vi "datatakersync_master.vi"() -> ()   [LabVIEW 2013, in "filenames.lvlib"]
doc: "This example demonstrates how to acquire a single buffer of voltage measurements using a DAQmx device.\n\nFor instructions on how to connect your signals to the DAQ device, refer to your device documentation."
uses:
  filenames.lvlib
  <vilib>/Analysis/3filter.llb/Filter Passband Type.ctl
  <vilib>/Utility/error.llb/DialogType.ctl
  <vilib>/DAQmx/write.llb/DAQmx Write (Analog 1D DBL 1Chan NSamp).vi
  <userlib>/Agilis Labview 7.1/AGILIS.llb/enter / leave remote mode.vi
  <vilib>/LabVIEW Hacker/LINX/Public/Peripherals/Analog/Analog Read 1 Chan.vi
  <vilib>/DAQmx/create/channels.llb/DAQmx Create Channel (AO-Voltage-Basic).vi
  <vilib>/DAQmx/configure/timing.llb/DAQmx Timing (Sample Clock).vi
  <vilib>/DAQmx/create/channels.llb/DAQmx Create Channel (AI-Voltage-Basic).vi
  <vilib>/DAQmx/configure/trigger.llb/DAQmx Start Trigger (Digital Edge).vi
  <vilib>/DAQmx/miscellaneous.llb/DAQmx Fill In Error Info.vi
  <resource>/objmgr/daqmx.rc
  <vilib>/LabVIEW Hacker/LINX/LVH-LINX.lvlib
  <vilib>/ptbypt/NI_PtbyPt.lvlib
  <vilib>/Analysis/NI_AALBase.lvlib
panel:
  in  "Jog during auto":bool=TRUE
  in  "Move Slide Back 3":bool
  in  "Move Slide  2":bool
  in  "Slide Jog Speed 2":i32(slide) scale=1.0..3.0
  in  "Stop Button":bool=TRUE
  in  "Use interferometer":bool=TRUE
  out "Motion Direction Indicator":bool
  out "Move Indicator":bool
  in  "Auto Move":bool=TRUE
  in  "Auto Motion Direction":bool
  in  "Tab Control":T1(tab)=enum."I/O"
  out "Indicator Pos 2":bool
  out "Indicator Pos 1":bool=TRUE
  in  "Go to 2":bool
  in  "Go to 1":bool
  in  "Cycles Between Movements":i32=1
  in  "Position 2":dbl=2.5
  in  "Position 1":dbl=-2.5
  out "Main Sig":dbl[][](graph)=[[-1.679588746006175], [-2.01550649520741]]
  out "Main Output":dbl(graph)=1.3000000000000012
  out "Displacement":dbl=1.3000000000000012 format="%#.3f"
  in  "Zero":bool
  in  "Go to Zero":bool
  in  "Automatic":bool=TRUE
  in  "Motion Direction":bool=TRUE
  in  "Manual Move":bool
  in  "Stop Movement":bool
  in  "Arduino Serial Port":refnum<visa-resource-name>="COM3"
  out "Device Name":string="Arduino Mega 2560"
  in  "Analog Channel":u8
  out "Filtered Signal":dbl(graph)=-1.679588746006175
  in  "filter type":T2=enum."Bandpass"
  in  "order":i32=2
  in  "initialize":bool
  in  "low cutoff freq: fl":dbl=0.45 format="%#_13g"
  out "Raw Signal":dbl(graph)=2.294921875
  in  "Positive Move Steps":i32=30
  in  "Controller Serial Port":u8=6
  in  "Negative Move Steps":i32=30
  in  "Move Period (ms)":u32=10
  in  "high cutoff freq: fh":dbl=1.0
  out "Input Signals":dbl[][](graph)=[[-1.679588746006175], [-2.01550649520741]]
  out "Stepped Signal":dbl(graph)=2.0
  in  "Fringe Counter Settings":T3={"Wavelength"=3.25e-07, "Divisions"=2.0, "Scaling Amplitude"=1.2, "Scaling Offset"=0.0} {"Scaling Offset" format="%0.2f"; "Scaling Amplitude" format="%0.2f"}
  out "Fringe Counter Output Signal":dbl[](graph)=[1.21875e-06]
  out "Relative Displacement":dbl=1.21875e-06
  out "Total Displacement":dbl(graph)=1.3000000000000012
  out "Reset Fringe Counter":bool
  out "Timeout":bool
  in  "Slide Jog Speed":i32(slide) scale=1.0..3.0
  in  "Move Slide":bool
  in  "Move Slide Back":bool
  in  "Error In":errorcluster
  in  "Turn off drive\nwhen flashing?":bool
  in  "set synth":bool
  in  "Sweep type":u16(ring)=1 items=["Chirp", "Single freq", "Both"]
  in  "VISA session":refnum<visa-resource-name>="GPIB0::10::INSTR"
  in  "Physical Channel synth_trigger":tag="Dev5/ao0"
  in  "Digitize on\nother comp?":bool
  in  "stop (F)":ext=100.0
  in  "start (F)":ext=100.0
  in  "Number of F Steps":i32=1
  in  "dc offset?":bool
  in  "volt_div":dbl=200.0
  in  "stop (V)":ext=0.05
  in  "start (V)":ext=0.05
  in  "Number of V Steps":i32=1
  out "error out":errorcluster
  in  "Physical Channel (drive signals)":tag="Dev5/ai0"
  out "Curr threshold":dbl
  in  "Stop threshold":dbl=0.05
  in  "Stop flashing below thresh":bool
  out "Pirani pressure (mbar)":string
  out "CC read error":errorcluster={"status"=FALSE, "code"=1073676294, "source"="VISA Read in read_pressure(SubVI).vi->hdf5(SubVI).vi->filenames.lvlib:datatakersync_master.vi"}
  out "CC pressure (mbar)":string
  out "Pirani read error":errorcluster={"status"=FALSE, "code"=1073676294, "source"="VISA Read in read_pressure(SubVI).vi->hdf5(SubVI).vi->filenames.lvlib:datatakersync_master.vi"}
  in  "# Pulses":i32=3
  in  "Output channel (for flashing)":tag="Dev4/ao0"
  in  "Number of cyles\nbetween flashes":i32=3
  in  "Flash lamp?":bool
  in  "File base name":string="urmbar_xyzcool_close"
  in  "Delay time between files(s)":dbl caption="Delay Time (s)"
  in  "Num files":i32=1000
  out "Temps (C):":dbl[](array[numeric])
  in  "VISA Refnum in":refnum<visa-resource-name>="GPIB0::19::INSTR"
  in  "Directory path":path=path "D:/Data/20150331/Bead6/tapping_close2"
  out "Waveform Graph":dbl[][](graph)
  in  "Number of Samples":i32=1000
  in  "Sample Rate":dbl=10000.0
  in  "Sample Clock Source":tag="/Dev2/PXI_Clk10"
  in  "Terminal Configuration":i32(ring)=-1 items=["default"=-1, "RSE"=10083, "NRSE"=10078, "Differential"=10106, "Pseudodifferential"=12529]
  in  "Max Voltage":dbl=10.0
  in  "Physical Channels (Position signals)":tag="Dev2/ai0:7"
  out "Actual Sample Rate":dbl=10000.0 format="%0.2f"
  # "Channel Settings"
  # "Acquired Data"
  # "Timing Settings"
  # "Flash Lamp Settings"
  # "Pressures and Temperatures"
  # "Logging Settings"
  # "."
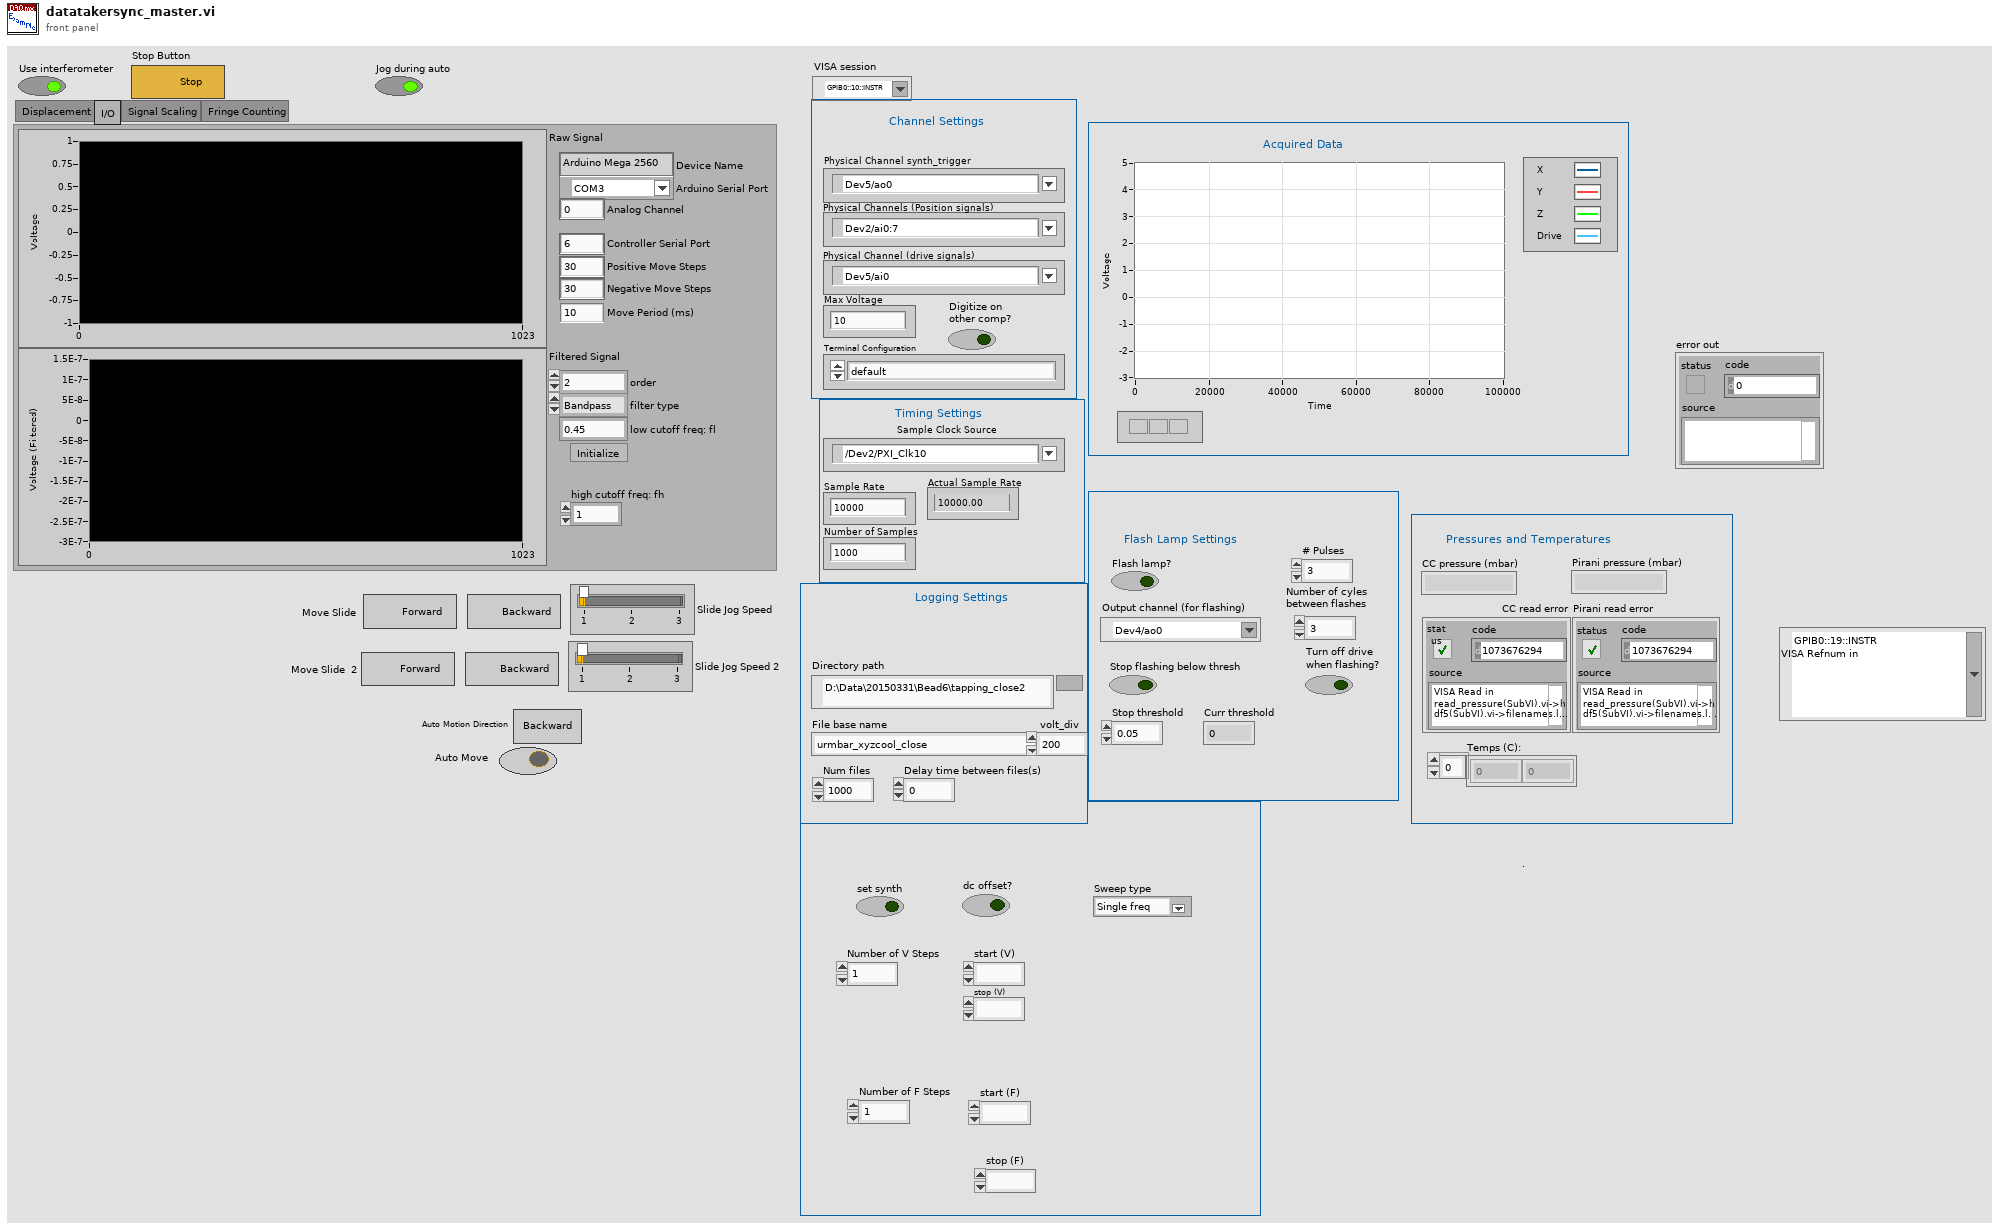
[diagram p1: front panel]
types:
  T1 = enum32{"Displacement", "I/O", "Signal Scaling", "Fringe Counting"}
  T2 = typedef "NI_AALBase.lvlib/Filter Passband Type.ctl" = enum32{"Lowpass", "Highpass", "Bandpass", "Bandstop"}
  T3 = cluster{"Wavelength":dbl, "Divisions":dbl, "Scaling Amplitude":dbl, "Scaling Offset":dbl}
  T4 = typedef "DialogType.ctl" = u16
  T5 = typedef "LVH-LINX.lvlib/LINX Ref.ctl" = cluster{"Platform":T6, "Interface":T7, "LINX Device Config":T8}
  T6 = typedef "LVH-LINX.lvlib/Platform.ctl" = enum16{"LINX", "myRIO"}
  T7 = typedef "LVH-LINX.lvlib/Interface.ctl" = enum16{"Serial", "TCP"}
  T8 = typedef "LVH-LINX.lvlib/Device.lvlib/LINX Device Config.ctl" = cluster{"Interface":T7, "COM Port":refnum<visa-resource-name>, "TCP Configuration":T9, "Device Family":T10, "Device ID":u8, "Device Name":string, "TCP Ref":refnum<k5>}
  T9 = typedef "LVH-LINX.lvlib/Device.lvlib/TCP Config.ctl" = cluster{"IP Address":string, "Port":u16}
  T10 = typedef "LVH-LINX.lvlib/Device Family.ctl" = enum8{"National Instruments", "Digilent", "Arduino"}
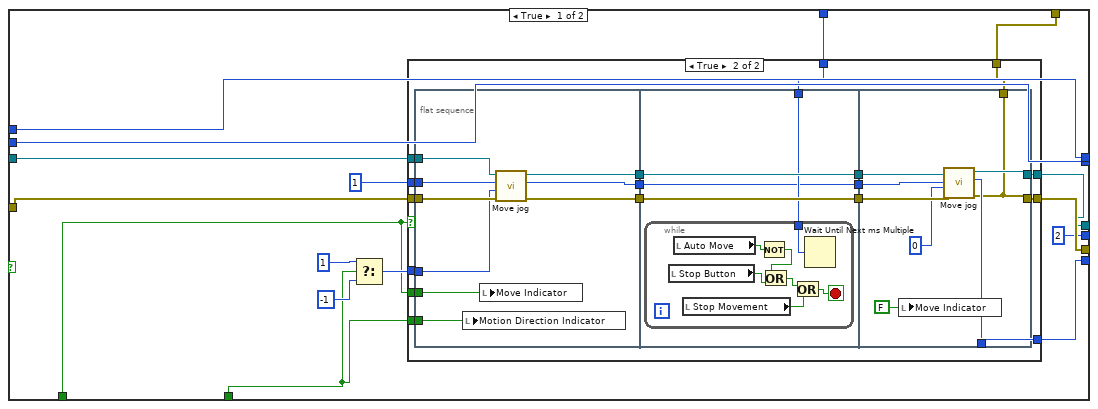
[diagram p3: hidden frame]
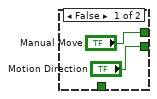
[diagram p5: hidden frame]
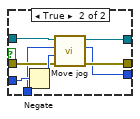
[diagram p6: hidden frame]
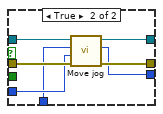
[diagram p7: hidden frame]
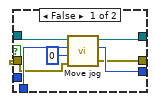
[diagram p8: hidden frame]
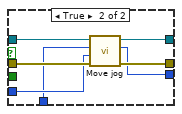
[diagram p9: hidden frame]
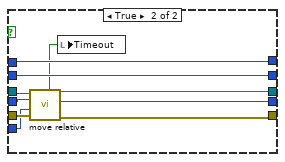
[diagram p10: hidden frame]
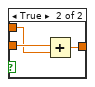
[diagram p13: hidden frame]
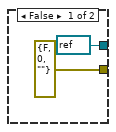
[diagram p14: hidden frame]
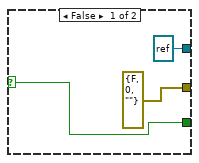
[diagram p17: hidden frame]
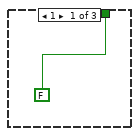
[diagram p18: hidden frame]
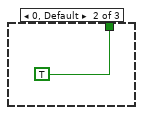
[diagram p19: hidden frame]
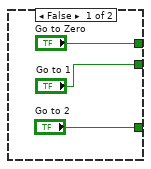
[diagram p20: hidden frame]
diagram:
  w10 = TRUE  # ID Query
  w46 = 10178 items=["Finite Samples"=10178, "Continuous Samples"=10123, "Hardware Timed Single Point"=12522]  # Sample Mode
  n1 = case shown="True" "set synth" {
    tunnel: w10 -> [_ w54]
    tunnel: [refnum<visa-resource-name> refnum ("dup VISA session") w51] -> w9
    tunnel: [errorcluster {"status"=FALSE, "code"=0, "source"=""} ("error out") w50] -> w8
    frame False {
    }
    frame True {
      n2 = call <vilib>:"ag33xxx - Initialize.vi"("ID Query (T: Check)"=w54, "Instrument Resource Name"="VISA session") -> ("error out"=w53:errorcluster, "dup VISA session"=w52:refnum<visa-resource-name>)  [unwired: 8 in]
      n3 = VISA Write(VISA resource name=w52, write buffer="SOUR:BM:NCYC INF;:SOUR:BM:PHAS 0;SOUR INT;:TRIG:SOUR EXT;:SOUR:BM:INT:RATE 1.000000;:BM:STAT ON;", error in (no error)=w53) -> (VISA resource name out=w51:refnum<visa-resource-name>, error out=w50:errorcluster)  [unwired: 1 out]
    }
  }
  n4 = call <vilib>:"Check if File or Folder Exists.vi"("path"="Directory path") -> ("file or folder exists?"=w36:bool, "dup path"=w35:path)  [unwired: 8 in, 1 out]
  n5 = case shown="False" w36 {
    tunnel: w35 -> [w57 w62]
    tunnel: [w56 w62] -> w34
    frame False {
      n6 = flat-sequence {
        tunnel: w57 -> [w61]
        tunnel: [w60] -> w56
        frame #0 {
          n7 = call "Create folder?"() -> ("OK"=w59:bool)  [unwired: 18 in, 1 out]
          n8 = Not(x=w59) -> (.not. x?=w58:bool)
          n9 = Stop(stop? (T)=w58) -> ()
        }
        frame #1 {
          n10 = Create Folder(path (use dialog)=w61) -> (created path=w60:path)  [unwired: 2 in, 2 out]
        }
      }
    }
    frame True {
    }
  }
  n11 = Subtract(x="stop (F)", y="start (F)") -> (x-y=w22:ext)
  n12 = Divide(x=w22, y="Number of F Steps") -> (x/y=w21:ext)
  n13 = Subtract(x="stop (V)", y="start (V)") -> (x-y=w29:ext)
  n14 = Multiply(x="Max Voltage", y=-1.0) -> (x*y=w39:dbl)
  n15 = Divide(x=w29, y="Number of V Steps") -> (x/y=w27:ext)
  n16 = case shown="True" "Digitize on\nother comp?" {
    selector: "Digitize on\nother comp?" -> [w63 w66]
    tunnel: [errorcluster {"status"=FALSE, "code"=0, "source"=""} ("error out") w69] -> w18
    tunnel: [refnum<k5> refnum ("connection ID") w68] -> w17
    tunnel: [w63 w66] -> w13
    frame False {
    }
    frame True {
      w70 = 60000  # timeout ms
      n17 = call <vilib>:"TCP Listen.vi"("timeout ms (wait forever: -1)"=w70, "port"=u16 6340) -> ("error out"=w69:errorcluster, "connection ID"=w68:refnum<k5>)  [unwired: 5 in, 3 out]
    }
  }
  n18 = local write "Automatic"(FALSE ("Go to Zero")) -> ()
  n19 = for {
    N: "Num files" -> [_]
    tunnel: w46 -> [w107]
    tunnel: "Physical Channels (Position signals)" -> [w106]
    tunnel: "Terminal Configuration" -> [w105]
    tunnel: "Sample Clock Source" -> [w104]
    tunnel: "Sample Rate" -> [w103]
    tunnel: "Number of Samples" -> [w102]
    tunnel: w39 -> [w101]
    tunnel: "Max Voltage" -> [w100]
    tunnel: w34 -> [w99]
    tunnel: "File base name" -> [w98]
    tunnel: "Output channel (for flashing)" -> [w97]
    tunnel: "Physical Channel (drive signals)" -> [w96]
    tunnel: "Number of V Steps" -> [w95]
    tunnel: w27 -> [w94]
    tunnel: "start (V)" -> [w93]
    tunnel: "Num files" -> [w92]
    tunnel: "set synth" -> [w91]
    tunnel: "volt_div" -> [w90]
    tunnel: w21 -> [w89]
    tunnel: "start (F)" -> [w88]
    tunnel: "Number of F Steps" -> [w87]
    tunnel: w18 -> [w86]
    tunnel: w17 -> [w85]
    tunnel: [w84] -> w16
    tunnel: [w83] -> w15
    tunnel: w13 -> [w82]
    tunnel: [w81] -> w12
    tunnel: "Physical Channel synth_trigger" -> [w80]
    tunnel: w9 -> [w79]
    tunnel: w8 -> [w78]
    tunnel: [w77] -> w7
    tunnel: [w76] -> w6
    tunnel: [w75] -> w5
    tunnel: "set synth" -> [w74]
    tunnel: "Sweep type" -> [w72]
    i -> [w71]
    n20 = case shown="2" w72 {
      tunnel: [FALSE TRUE w110] -> w73
      tunnel: w71 -> [_ _ w114]
      frame 1 {
      }
      frame 0, Default {
      }
      frame 2 {
        n21 = Quotient & Remainder(x=w114, y=2) -> (x-y*floor(x/y)=w112:i32)  [unwired: 1 out]
        n22 = Equal?(x=w112, y=0) -> (x = y?=w110:bool)
      }
    }
    n23 = for {
      N: w95 -> [_]
      tunnel: w107 -> [w151]
      tunnel: w106 -> [w150]
      tunnel: w105 -> [w149]
      tunnel: w104 -> [w148]
      tunnel: w103 -> [w147]
      tunnel: w102 -> [w146]
      tunnel: w101 -> [w145]
      tunnel: w100 -> [w144]
      tunnel: w99 -> [w143]
      tunnel: w98 -> [w142]
      tunnel: w97 -> [w141]
      tunnel: w96 -> [w140]
      tunnel: w94 -> [w139]
      tunnel: w93 -> [w138]
      tunnel: w71 -> [w136]
      tunnel: w92 -> [w135]
      tunnel: w91 -> [w134]
      tunnel: w90 -> [w133]
      tunnel: w89 -> [w132]
      tunnel: w88 -> [w131]
      tunnel: w87 -> [w130]
      tunnel: w73 -> [w129]
      tunnel: w86 -> [w128]
      tunnel: w85 -> [w127]
      tunnel: [w126] -> w84
      tunnel: [w125] -> w83
      tunnel: w82 -> [w124]
      tunnel: [w123] -> w81
      tunnel: w80 -> [w122]
      tunnel: w79 -> [w121]
      tunnel: w78 -> [w120]
      tunnel: [w119] -> w77
      tunnel: [w118] -> w76
      tunnel: [w117] -> w75
      tunnel: w74 -> [w116]
      tunnel: w71 -> [w115]
      i -> [w137]
      n24 = for {
        N: w130 -> [_]
        tunnel: w151 -> [w284]
        tunnel: w150 -> [w283]
        tunnel: w149 -> [w282]
        tunnel: w148 -> [w281]
        tunnel: w147 -> [w209]
        tunnel: w146 -> [w280]
        tunnel: w145 -> [w279]
        tunnel: w144 -> [w278]
        tunnel: w143 -> [w277]
        tunnel: w142 -> [w276]
        tunnel: w141 -> [w275]
        tunnel: w140 -> [w274]
        tunnel: w139 -> [w273]
        tunnel: w138 -> [w271]
        tunnel: w137 -> [w269]
        tunnel: w136 -> [w268]
        tunnel: w135 -> [w237]
        tunnel: w134 -> [w267]
        tunnel: w133 -> [w266]
        tunnel: w132 -> [w262]
        tunnel: w131 -> [w261]
        tunnel: w129 -> [w259]
        tunnel: w128 -> [w258]
        tunnel: w127 -> [w257]
        tunnel: [w256] -> w126
        tunnel: [w255] -> w125
        tunnel: w124 -> [w254]
        tunnel: [w253] -> w123
        tunnel: w122 -> [w208]
        tunnel: w121 -> [w204]
        tunnel: w120 -> [w203]
        tunnel: [w199] -> w119
        tunnel: [w195] -> w118
        tunnel: [w194] -> w117
        tunnel: w116 -> [w190]
        tunnel: w115 -> [w152]
        i -> [w260]
        n25 = Multiply(x=w262, y=w260) -> (x*y=w263:ext)
        n26 = Add(x=w261, y=w263) -> (x+y=w264:ext)
        n27 = Multiply(x=w269, y=w273) -> (x*y=w272:ext)
        n28 = Add(x=w271, y=w272) -> (x+y=w270:ext)
        n29 = flat-sequence {
          tunnel: w190 -> [w292]
          tunnel: w203 -> [w293]
          tunnel: w204 -> [w294]
          tunnel: w208 -> [w295]
          tunnel: w254 -> [w296]
          tunnel: w257 -> [w297]
          tunnel: w258 -> [w298]
          tunnel: w259 -> [w299]
          tunnel: "dc offset?" -> [w300]
          tunnel: w267 -> [w301]
          tunnel: w268 -> [w302]
          tunnel: w270 -> [w303]
          tunnel: w270 -> [w304]
          tunnel: w264 -> [w305]
          tunnel: w274 -> [w306]
          tunnel: w275 -> [w307]
          tunnel: w276 -> [w308]
          tunnel: w277 -> [w309]
          tunnel: w278 -> [w310]
          tunnel: w279 -> [w311]
          tunnel: w281 -> [w312]
          tunnel: w282 -> [w313]
          tunnel: w283 -> [w314]
          tunnel: [w314] -> w175
          tunnel: [w313] -> w174
          tunnel: [w312] -> w173
          tunnel: [w311] -> w172
          tunnel: [w310] -> w171
          tunnel: [w309] -> w170
          tunnel: [w308] -> w169
          tunnel: [w307] -> w168
          tunnel: [w306] -> w167
          tunnel: [w305] -> w166
          tunnel: [w304] -> w165
          tunnel: [w303] -> w164
          tunnel: [w302] -> w163
          tunnel: [w301] -> w162
          tunnel: [w300] -> w161
          tunnel: [w299] -> w160
          tunnel: [w298] -> w159
          tunnel: [w297] -> w158
          tunnel: [w296] -> w157
          tunnel: [w295] -> w156
          tunnel: [w294] -> w155
          tunnel: [w293] -> w154
          tunnel: [w292] -> w153
          tunnel: w152 -> [w285]
          tunnel: [w391] -> w241
          tunnel: [w390] -> w242
          tunnel: [w389] -> w243
          tunnel: [w388] -> w244
          tunnel: [w387] -> w245
          tunnel: [w386] -> w246
          tunnel: [w385] -> w247
          tunnel: [w384] -> w248
          tunnel: [w383] -> w249
          tunnel: [w381] -> w250
          tunnel: [w380] -> w251
          tunnel: [w379] -> w252
          tunnel: [w377] -> w240
          tunnel: [w376] -> w239
          tunnel: [w375] -> w238
          tunnel: [w374] -> w207
          tunnel: [w371] -> w202
          tunnel: [w370] -> w198
          tunnel: [w369] -> w191
          tunnel: [w368] -> w186
          tunnel: [w367] -> w185
          tunnel: [w366] -> w180
          tunnel: w175 -> [w391]
          tunnel: w174 -> [w390]
          tunnel: w173 -> [w389]
          tunnel: w172 -> [w388]
          tunnel: w171 -> [w387]
          tunnel: w170 -> [w386]
          tunnel: w169 -> [w385]
          tunnel: w168 -> [w384]
          tunnel: w167 -> [w383]
          tunnel: w166 -> [w381]
          tunnel: w165 -> [w382]
          tunnel: w164 -> [w380]
          tunnel: w163 -> [w379]
          tunnel: w162 -> [w378]
          tunnel: w161 -> [w366]
          tunnel: w160 -> [w368]
          tunnel: w159 -> [w377]
          tunnel: w158 -> [w376]
          tunnel: w157 -> [w375]
          tunnel: w156 -> [w374]
          tunnel: w155 -> [w373]
          tunnel: w154 -> [w372]
          tunnel: w153 -> [w369]
          tunnel: w252 -> [w443]
          tunnel: w251 -> [w413]
          tunnel: w250 -> [w448]
          tunnel: [w448] -> w236
          tunnel: w249 -> [w457]
          tunnel: [w457] -> w234
          tunnel: w248 -> [w456]
          tunnel: [w456] -> w232
          tunnel: w247 -> [w422]
          tunnel: w246 -> [w424]
          tunnel: w245 -> [w455]
          tunnel: [w455] -> w229
          tunnel: w244 -> [w454]
          tunnel: [w454] -> w227
          tunnel: w243 -> [w453]
          tunnel: [w453] -> w225
          tunnel: w242 -> [w452]
          tunnel: [w452] -> w223
          tunnel: w241 -> [w451]
          tunnel: [w451] -> w221
          tunnel: w240 -> [w433]
          tunnel: [w430] -> w219
          tunnel: w239 -> [w434]
          tunnel: [w431] -> w217
          tunnel: w238 -> [w432]
          tunnel: [w429] -> w215
          tunnel: [w449] -> w213
          tunnel: w237 -> [w446]
          tunnel: [w443] -> w211
          tunnel: w207 -> [w428]
          tunnel: [w428] -> w205
          tunnel: w202 -> [w427]
          tunnel: [w427] -> w200
          tunnel: w198 -> [w426]
          tunnel: [w426] -> w196
          tunnel: [w425] -> w193
          tunnel: w191 -> [w425]
          tunnel: [w424] -> w189
          tunnel: [w423] -> w188
          tunnel: w186 -> [w416]
          tunnel: w185 -> [w415]
          tunnel: [w416] -> w183
          tunnel: [w415] -> w182
          tunnel: w180 -> [w414]
          tunnel: [w414] -> w179
          tunnel: [w413] -> w177
          tunnel: w236 -> [w515]
          tunnel: [w515] -> w235
          tunnel: w234 -> [w514]
          tunnel: [w514] -> w233
          tunnel: w232 -> [w513]
          tunnel: [w513] -> w231
          tunnel: [w512] -> w230
          tunnel: w229 -> [w511]
          tunnel: [w511] -> w228
          tunnel: w227 -> [w510]
          tunnel: [w510] -> w226
          tunnel: w225 -> [w509]
          tunnel: [w509] -> w224
          tunnel: w223 -> [w508]
          tunnel: [w508] -> w222
          tunnel: w221 -> [w502]
          tunnel: [w502] -> w220
          tunnel: w219 -> [w507]
          tunnel: [w507] -> w218
          tunnel: w217 -> [w506]
          tunnel: [w506] -> w216
          tunnel: w215 -> [w505]
          tunnel: [w505] -> w214
          tunnel: w213 -> [w504]
          tunnel: [w504] -> w212
          tunnel: w211 -> [w503]
          tunnel: [w503] -> w210
          tunnel: [w501] -> w206
          tunnel: w205 -> [w501]
          tunnel: [w500] -> w201
          tunnel: w200 -> [w500]
          tunnel: [w499] -> w197
          tunnel: w196 -> [w499]
          tunnel: w193 -> [w498]
          tunnel: [w498] -> w192
          tunnel: w189 -> [w512]
          tunnel: w188 -> [w497]
          tunnel: [w497] -> w187
          tunnel: [w496] -> w184
          tunnel: w183 -> [w496]
          tunnel: w182 -> [w495]
          tunnel: [w495] -> w181
          tunnel: w179 -> [w494]
          tunnel: [w494] -> w178
          tunnel: w177 -> [w493]
          tunnel: [w493] -> w176
          tunnel: w284 -> [w618]
          tunnel: w209 -> [w538]
          tunnel: w280 -> [w615]
          tunnel: w266 -> [w568]
          tunnel: w235 -> [w528]
          tunnel: w233 -> [w611]
          tunnel: w231 -> [w612]
          tunnel: w230 -> [w562]
          tunnel: w228 -> [w613]
          tunnel: w226 -> [w614]
          tunnel: w224 -> [w560]
          tunnel: w222 -> [w616]
          tunnel: w220 -> [w617]
          tunnel: w218 -> [w564]
          tunnel: w216 -> [w565]
          tunnel: [w564] -> w256
          tunnel: [w565] -> w255
          tunnel: w214 -> [w563]
          tunnel: [w563] -> w253
          tunnel: w212 -> [w567]
          tunnel: w210 -> [w566]
          tunnel: w206 -> [w561]
          tunnel: w201 -> [w523]
          tunnel: [w522] -> w199
          tunnel: w197 -> [w527]
          tunnel: [w521] -> w195
          tunnel: [w546] -> w194
          tunnel: w192 -> [w546]
          tunnel: w187 -> [w545]
          tunnel: w184 -> [w526]
          tunnel: w181 -> [w525]
          tunnel: w178 -> [w524]
          tunnel: w176 -> [w520]
          frame #0 {
            n30 = case shown="True" "Automatic" {
              tunnel: w285 -> [_ w325]
              tunnel: ["Go to Zero" FALSE ("Go to Zero")] -> w288
              tunnel: ["Go to 1" w319] -> w289
              tunnel: ["Go to 2" w320] -> w290
              frame False {
              }
              frame True {
                n31 = Quotient & Remainder(x=w325, y="Cycles Between Movements") -> (x-y*floor(x/y)=w323:i32, floor(x/y)=w321:i32)
                n32 = Equal To 0?(x=w323) -> (x = 0?=w322:bool)
                n33 = case shown="True" w322 {
                  tunnel: w321 -> [_ w331]
                  tunnel: [w326 w328] -> w320
                  tunnel: [w326 w327] -> w319
                  frame False {
                    w326 = FALSE
                  }
                  frame True {
                    n34 = Quotient & Remainder(x=w331, y=2) -> (x-y*floor(x/y)=w329:i32)  [unwired: 1 out]
                    n35 = Equal To 0?(x=w329) -> (x = 0?=w327:bool)
                    n36 = Not(x=w327) -> (.not. x?=w328:bool)
                  }
                }
              }
            }
            n37 = local read "Displacement"() -> (w287:dbl)
            n38 = for {
              N: 3 -> [_]
              tunnel: w288 -> [w337]
              tunnel: w289 -> [w334]
              tunnel: w290 -> [w333]
              tunnel: w287 -> [w335]
              i -> [w338]
              n39 = case shown="2" w338 {
                tunnel: w337 -> [w361 _ _]
                tunnel: w334 -> [_ w363 _]
                tunnel: w333 -> [_ _ w365]
                tunnel: [w361 w363 w365] -> w332
                tunnel: [0.0 ("Position 2") "Position 1" "Position 2"] -> w336
                frame 0, Default {
                }
                frame 1 {
                }
                frame 2 {
                }
              }
              n40 = case shown="True" w332 {
                tunnel: w336 -> [_ w345]
                tunnel: w335 -> [_ w344]
                tunnel: w334 -> [_ w340]
                tunnel: w333 -> [_ w341]
                tunnel: w332 -> [_ w339]
                frame False {
                }
                frame True {
                  n41 = Greater?(x=w345, y=w344) -> (0:w343:bool)
                  n42 = local write "Auto Motion Direction"(w343) -> ()
                  n43 = local write "Auto Move"(w339) -> ()
                  n44 = while {
                    tunnel: w345 -> [w346]
                    tunnel: w343 -> [w358]
                    tunnel: w341 -> [w355]
                    tunnel: w340 -> [w354]
                    tunnel: [FALSE] -> w342
                    stop <- w351 stop-if-true
                    n45 = local read "Displacement"() -> (w347:dbl)
                    n46 = Not Equal?(x=w347, y=w346) -> (x != y?=w348:bool)
                    n47 = Greater?(x=w346, y=w347) -> (0:w359:bool)
                    n48 = Equal?(x=w359, y=w358) -> (x = y?=w353:bool)
                    n49 = And(x=w348, y=w353) -> (x .and. y?=w349:bool)
                    n50 = And(x=w354, y=w349) -> (x .and. y?=→"Indicator Pos 1":bool)
                    n51 = And(x=w355, y=w349) -> (x .and. y?=→"Indicator Pos 2":bool)
                    n52 = Compound Arithmetic op=OR(invert w349, "Stop Movement") -> (w351:bool)
                  }
                  n53 = local write "Auto Move"(w342) -> ()
                }
              }
            }
          }
          frame #1 {
            n54 = case shown="True" w378 {
              tunnel: w382 -> [_ w403]
              tunnel: w381 -> [_ w402]
              tunnel: w366 -> [_ w401]
              tunnel: w368 -> [_ w400]
              tunnel: w373 -> [w393 w399]
              tunnel: w372 -> [w394 w398]
              tunnel: [w394 w397] -> w371
              tunnel: [w393 w396] -> w370
              tunnel: ["no_synth" ("User Def. Wfm Name") w395] -> w367
              frame False {
              }
              frame True {
                n55 = flat-sequence {
                  tunnel: w403 -> [w412]
                  tunnel: w402 -> [w411]
                  tunnel: w401 -> [w410]
                  tunnel: w400 -> [w409]
                  tunnel: w399 -> [w408]
                  tunnel: w398 -> [w407]
                  tunnel: [w406] -> w397
                  tunnel: [w405] -> w396
                  tunnel: [w404] -> w395
                  frame #0 {
                    w404 = "RANDFREQ" ("User Def. Wfm Name")
                    n56 = call "synth_set(SubVI).vi"("dc offset?"=w410, "error in (no error)"=w407, "User Def. Wfm Name"=w404, "chirp?"=w409, "VISA session"=w408, "amplitude (V)"=w412, "frequency (Hz)"=w411) -> ("dup VISA session"=w405:refnum<visa-resource-name>, "error out"=w406:errorcluster)  [unwired: 3 in]
                  }
                  frame #1 {
                    n57 = call "Time Delay2"() -> ()  [unwired: 11 in, 1 out]
                  }
                }
              }
            }
          }
          frame #2 {
            n58 = Multiply(x=w413, y=ext 1000.0) -> (x*y=w449:ext)
            n59 = Number To Decimal String(number=w449) -> (decimal integer string=w420:string)  [unwired: 1 in]
            n60 = Number To Decimal String(number=w448) -> (decimal integer string=w418:string)  [unwired: 1 in]
            n61 = case shown="True" w416 {
              tunnel: [w464 w465] -> w444
              tunnel: w422 -> [w463 w470]
              tunnel: "_" ("string") -> [w462 w469]
              tunnel: w420 -> [w461 w468]
              tunnel: "mV_" ("string") -> [w460 w467]
              tunnel: w418 -> [w459 _]
              tunnel: "Hz" ("string") -> [w458 _]
              tunnel: w415 -> [_ w466]
              frame False {
                n62 = Concatenate Strings(w463, w462, w461, w460, w459, w458) -> (w464:string)
              }
              frame True {
                n63 = Concatenate Strings(w470, w469, w468, w467, w466) -> (w465:string)
              }
            }
            n64 = Greater?(x=w446, y=1) -> (0:w445:bool)
            n65 = case shown="False" w445 {
              tunnel: w443 -> [_ w492]
              tunnel: [w486 w491] -> w442
              tunnel: w444 -> [w485 w490]
              frame False {
                n66 = Concatenate Strings(w485, ".h5" ("string")) -> (w486:string)
              }
              frame True {
                n67 = Number To Decimal String(number=w492) -> (decimal integer string=w488:string)  [unwired: 1 in]
                n68 = Concatenate Strings(w490, "_" ("string"), w488, ".h5" ("string")) -> (w491:string)
              }
            }
            n69 = Build Path(base path=w424, name or relative path=w442) -> (appended path=w423:path)
            n70 = Path To String(path=w423) -> (string=w439:string)
            n71 = Search and Replace String(input string=w439, search string=".h5", replace string="_drive.h5" ("substring (\"\")")) -> (result string=w438:string)  [unwired: 5 in, 3 out]
            n72 = Search and Replace String(input string=w438, search string="D:", replace string="C:" ("replace string (\"\")")) -> (result string=w435:string)  [unwired: 5 in, 3 out]
            n73 = case shown="True" w432 {
              selector: w432 -> [w471 w474]
              tunnel: w433 -> [w472 w483]
              tunnel: w434 -> [w473 w482]
              tunnel: w435 -> [_ w481]
              tunnel: [w472 w476] -> w430
              tunnel: [w473 w475] -> w431
              tunnel: [w471 w474] -> w429
              frame False {
              }
              frame True {
                n74 = String Length(string=w481) -> (length=w478:i32)
                n75 = Type Cast(x=w478) -> (*(type *) &x=w477:string)  [unwired: 1 in]
                n76 = TCP Write(connection ID=w482, data in=w477, error in (no error)=w483) -> (connection ID out=w480:refnum<k5>, error out=w479:errorcluster)  [unwired: 1 in, 1 out]
                n77 = TCP Write(connection ID=w480, data in=w481, error in (no error)=w479) -> (connection ID out=w475:refnum<k5>, error out=w476:errorcluster)  [unwired: 1 in, 1 out]
              }
            }
          }
          frame #3 {
            n78 = call "Time Delay3"() -> ()  [unwired: 11 in, 1 out]
          }
          frame #4 {
            w552 = T4 3 items=["no dialog", "OK message", "continue or stop message", "OK message + warnings", "continue/stop + warnings"] ("type of dialog (OK msg:1)")
            w580 = T4 3 items=["no dialog", "OK message", "continue or stop message", "OK message + warnings", "continue/stop + warnings"] ("type of dialog (OK msg:1)")
            w603 = T4 3 items=["no dialog", "OK message", "continue or stop message", "OK message + warnings", "continue/stop + warnings"] ("type of dialog (OK msg:1)")
            # "Acquire Data"
            # "Acquire Data"
            n79 = flat-sequence {
              tunnel: w538 -> [w644]
              tunnel: w560 -> [w648]
              tunnel: w561 -> [w649]
              tunnel: "# Pulses" -> [w646]
              tunnel: w516 -> [w647]
              tunnel: w611 -> [w650]
              tunnel: w612 -> [w645]
              tunnel: w613 -> [w651]
              tunnel: w614 -> [w652]
              tunnel: w615 -> [w653]
              tunnel: w616 -> [w654]
              tunnel: w617 -> [w655]
              tunnel: [w655] -> w537
              tunnel: [w654] -> w536
              tunnel: [w653] -> w535
              tunnel: [w652] -> w534
              tunnel: [w651] -> w533
              tunnel: [w650] -> w532
              tunnel: [w649] -> w531
              tunnel: [w648] -> w530
              tunnel: [w644] -> w529
              tunnel: w528 -> [w642]
              tunnel: w527 -> [w641]
              tunnel: w526 -> [w640]
              tunnel: w525 -> [w639]
              tunnel: w524 -> [w638]
              tunnel: w523 -> [w637]
              tunnel: [w634] -> w522
              tunnel: [w631] -> w521
              tunnel: w520 -> [w626]
              tunnel: w517 -> [w621]
              tunnel: w618 -> [w751]
              tunnel: [w744] -> w602
              tunnel: [w731] -> w590
              tunnel: [w730] -> w589
              tunnel: [w729] -> w588
              tunnel: [w728] -> w587
              tunnel: [w711] -> w559
              tunnel: [w710] -> w556
              tunnel: w537 -> [w750]
              tunnel: w536 -> [w749]
              tunnel: w535 -> [w748]
              tunnel: w534 -> [w747]
              tunnel: w533 -> [w746]
              tunnel: w532 -> [w745]
              tunnel: w531 -> [w721]
              tunnel: w530 -> [w715]
              tunnel: w529 -> [w709]
              frame #0 {
                n80 = flat-sequence {
                  tunnel: w646 -> [w665]
                  tunnel: [w665] -> w643
                  tunnel: w642 -> [w659]
                  tunnel: w641 -> [w664]
                  tunnel: w640 -> [w660]
                  tunnel: w639 -> [w658]
                  tunnel: w638 -> [w657]
                  tunnel: w637 -> [w663]
                  tunnel: [w662] -> w635
                  tunnel: [w661] -> w632
                  tunnel: [w660] -> w630
                  tunnel: [w659] -> w628
                  tunnel: [w658] -> w625
                  tunnel: [w657] -> w623
                  tunnel: w621 -> [w656]
                  tunnel: [w656] -> w619
                  tunnel: w647 -> [w687]
                  tunnel: w645 -> [w685]
                  tunnel: w644 -> [w684]
                  tunnel: w643 -> [w686]
                  tunnel: [w683] -> w636
                  tunnel: w635 -> [w683]
                  tunnel: [w682] -> w633
                  tunnel: w632 -> [w682]
                  tunnel: w630 -> [w681]
                  tunnel: [w681] -> w629
                  tunnel: w628 -> [w680]
                  tunnel: [w680] -> w627
                  tunnel: w625 -> [w679]
                  tunnel: [w679] -> w624
                  tunnel: w623 -> [w678]
                  tunnel: [w678] -> w622
                  tunnel: [w677] -> w620
                  tunnel: w619 -> [w677]
                  tunnel: w636 -> [w696]
                  tunnel: [w694] -> w634
                  tunnel: w633 -> [w697]
                  tunnel: [w695] -> w631
                  tunnel: w629 -> [w693]
                  tunnel: w627 -> [w692]
                  tunnel: w626 -> [w691]
                  tunnel: w624 -> [w690]
                  tunnel: w622 -> [w689]
                  tunnel: w620 -> [w688]
                  frame #0 {
                    n81 = case shown="True" w656 {
                      tunnel: w664 -> [w667 w675]
                      tunnel: w663 -> [w666 w674]
                      tunnel: [w666 w673] -> w662
                      tunnel: [w667 w672] -> w661
                      tunnel: w660 -> [_ w671]
                      tunnel: w659 -> [_ w670]
                      tunnel: w658 -> [_ w669]
                      tunnel: w657 -> [_ w668]
                      frame False {
                      }
                      frame True {
                        n82 = call "synth_set(SubVI).vi"("dc offset?"=w668, "error in (no error)"=w674, "User Def. Wfm Name"=w669, "chirp?"=w671, "VISA session"=w675, "amplitude (V)"=ext 0.05, "frequency (Hz)"=w670) -> ("dup VISA session"=w672:refnum<visa-resource-name>, "error out"=w673:errorcluster)  [unwired: 3 in]
                        n83 = call "Time Delay4"() -> ()  [unwired: 11 in, 1 out]
                      }
                    }
                  }
                  frame #1 {
                    n84 = call "flasher(SubVI).vi"("Sample Rate"=w684, "# Pulses"=w686, "Boolean"=w687, "Output channel (for flashing)"=w685) -> ()  [unwired: 8 in]
                  }
                  frame #2 {
                    n85 = case shown="True" w688 {
                      tunnel: w697 -> [w698 w708]
                      tunnel: w696 -> [w699 w707]
                      tunnel: [w698 w706] -> w695
                      tunnel: [w699 w705] -> w694
                      tunnel: w693 -> [_ w704]
                      tunnel: w692 -> [_ w703]
                      tunnel: w691 -> [_ w702]
                      tunnel: w690 -> [_ w701]
                      tunnel: w689 -> [_ w700]
                      frame False {
                      }
                      frame True {
                        n86 = call "synth_set(SubVI).vi"("dc offset?"=w700, "error in (no error)"=w707, "User Def. Wfm Name"=w701, "chirp?"=w704, "VISA session"=w708, "amplitude (V)"=w702, "frequency (Hz)"=w703) -> ("dup VISA session"=w706:refnum<visa-resource-name>, "error out"=w705:errorcluster)  [unwired: 3 in]
                        n87 = call "Time Delay5"() -> ()  [unwired: 11 in, 1 out]
                      }
                    }
                  }
                }
              }
              frame #1 {
                w716 = 10000000.0 ("RefClk.Rate")
                # "Trigger Settings"
                # "Timing Settings"
                # "Channel Settings"
                n88 = call-poly <vilib>:"DAQmx Create Virtual Channel.vi"("maximum value"=w746, "minimum value"=w747, "input terminal configuration"=w749, "physical channels"=w745) -> ("task out"=w741:refnum<k21>)  [unwired: 10 in, 1 out]
                n89 = call-poly <vilib>:"DAQmx Create Virtual Channel.vi"("maximum value"=w746, "minimum value"=w747, "input terminal configuration"=w749, "physical channels"=w750) -> ("task out"=w743:refnum<k21>, "error out"=w742:errorcluster)  [unwired: 10 in]
                n90 = call-poly <vilib>:"DAQmx Create Virtual Channel.vi"("physical channels"=w721) -> ("task out"=w720:refnum<k21>, "error out"=w718:errorcluster)  [unwired: 13 in]
                n91 = call-poly <vilib>:"DAQmx Timing.vi"("task/channels in"=w741, "sample mode"=w751, "samples per channel"=w748, "rate"=w709) -> ("task out"=w738:refnum<k21>, "error out"=w737:errorcluster)  [unwired: 10 in]
                n92 = call-poly <vilib>:"DAQmx Timing.vi"("task/channels in"=w720, "rate"=w709, "error in"=w718) -> ("task out"=w719:refnum<k21>, "error out"=w717:errorcluster)  [unwired: 11 in]
                n93 = call-poly <vilib>:"DAQmx Timing.vi"("task/channels in"=w743, "sample mode"=w751, "samples per channel"=w748, "rate"=w709, "error in"=w742) -> ("task out"=w740:refnum<k21>, "error out"=w739:errorcluster)  [unwired: 9 in]
                n94 = property class="DAQmx Timing"(reference=w738, error in=w737, "More:Reference Clock:Source"=w715, "More:Reference Clock:Rate"=w716) -> (reference out=w733:refnum<k21>, error out=w732:errorcluster)
                n95 = property class="DAQmx Timing"(reference=w740, error in=w739, "More:Reference Clock:Source"=w715, "More:Reference Clock:Rate"=w716) -> (reference out=w736:refnum<k21>, error out=w735:errorcluster)
                n96 = property class="DAQmx Timing"(reference=w719, error in=w717, "More:Reference Clock:Source"=w715, "More:Reference Clock:Rate"=w716) -> (reference out=w713:refnum<k21>, error out=w714:errorcluster)
                n97 = property class="DAQmx Timing"(reference=w736, error in=w735) -> (reference out=w727:refnum<k21>, error out=w725:errorcluster, "SampClk.Rate"=w744:dbl)
                "Actual Sample Rate" <- w744
                n98 = property class="DAQmx Export Signal"(reference=w727, error in=w725, "StartTrig.OutputTerm"=tag "/Dev2/PFI1", "StartTrig.OutputTerm"=tag "/Dev2/PFI0" ("10MHzRefClk.OutputTerm")) -> (reference out=w726:refnum<k21>, error out=w724:errorcluster)
                n99 = call "Get Full Terminal Name.vi"("error in (no error)"=w724, "Local Terminal Name"="ai/StartTrigger", "task/channels in"=w726) -> ("error out"=w730:errorcluster, "Terminal Name with Device Prefix"=w712:tag, "task out"=w731:refnum<k21>)  [unwired: 6 in]
                n100 = call-poly <vilib>:"DAQmx Trigger.vi"("task/channels in"=w733, "source"=w712, "error in"=w732) -> ("task out"=w729:refnum<k21>, "error out"=w728:errorcluster)  [unwired: 11 in]
                n101 = call-poly <vilib>:"DAQmx Trigger.vi"("task/channels in"=w713, "source"=w712, "error in"=w714) -> ("task out"=w710:refnum<k21>, "error out"=w711:errorcluster)  [unwired: 11 in]
              }
            }
            n102 = call "threshold_stop(SubVI).vi"("Stop threshold"="Stop threshold", "Stop flashing below thresh"="Stop flashing below thresh", "dup path"=w562) -> ("Curr threshold"=→"Curr threshold":dbl, "Boolean"=w594:bool)  [unwired: 7 in]
            n103 = call "flash_cycle(SubVI).vi"("Boolean in"=w594, "Number of cyles\nbetween flashes"="Number of cyles\nbetween flashes", "Numeric"=w566, "Flash lamp?"="Flash lamp?") -> ("Boolean out"=w516:bool)  [unwired: 7 in]
            n104 = And(x="Turn off drive\nwhen flashing?", y=w516) -> (x .and. y?=w517:bool)
            n105 = Select(t="# Pulses", s=w516, f=0) -> (s? t:f=w591:i32)
            n106 = flat-sequence {
              tunnel: w556 -> [w752]
              tunnel: w559 -> [w753]
              tunnel: w587 -> [w754]
              tunnel: w588 -> [w755]
              tunnel: w589 -> [w756]
              tunnel: w590 -> [w757]
              tunnel: [w757] -> w544
              tunnel: [w756] -> w543
              tunnel: [w755] -> w542
              tunnel: [w754] -> w541
              tunnel: [w753] -> w540
              tunnel: [w752] -> w539
              tunnel: [w773] -> w610
              tunnel: [w772] -> w609
              tunnel: [w771] -> w608
              tunnel: [w770] -> w607
              tunnel: [w769] -> w558
              tunnel: [w768] -> w557
              tunnel: w544 -> [w773]
              tunnel: w543 -> [w772]
              tunnel: w542 -> [w775]
              tunnel: w541 -> [w774]
              tunnel: w540 -> [w762]
              tunnel: w539 -> [w764]
              tunnel: [w782] -> w600
              tunnel: [w780] -> w601
              tunnel: w610 -> [w783]
              tunnel: w609 -> [w781]
              tunnel: [w779] -> w586
              tunnel: w608 -> [w779]
              tunnel: [w778] -> w585
              tunnel: w607 -> [w778]
              tunnel: w558 -> [w777]
              tunnel: [w777] -> w549
              tunnel: w557 -> [w776]
              tunnel: [w776] -> w548
              frame #0 {
              }
              frame #1 {
                n107 = Initialize Array(0.0 ("element"), 100 ("dimension size")) -> (w760:dbl[])
                n108 = Replace Array Subset(array=w760, new element=5.0 ("new element/subarray"), index=1) -> (w765:dbl[])
                n109 = call-poly <vilib>:"DAQmx Write.vi"("task/channels in"=w764, "data"=w765, "error in"=w762) -> ("task out"=w763:refnum<k21>, "error out"=w761:errorcluster)  [unwired: 10 in, 1 out]
                n110 = call <vilib>:"DAQmx Start Task.vi"("task/channels in"=w775, "error in"=w774) -> ("task out"=w771:refnum<k21>, "error out"=w770:errorcluster)  [unwired: 12 in]
                n111 = call <vilib>:"DAQmx Start Task.vi"("task/channels in"=w763, "error in"=w761) -> ("task out"=w769:refnum<k21>, "error out"=w768:errorcluster)  [unwired: 12 in]
              }
              frame #2 {
                n112 = call <vilib>:"DAQmx Start Task.vi"("task/channels in"=w783, "error in"=w781) -> ("task out"=w782:refnum<k21>, "error out"=w780:errorcluster)  [unwired: 12 in]
              }
            }
            n113 = call "hdf5(SubVI).vi"("Refnum in"=w600, "VISA Refnum in"="VISA Refnum in", "appended path"=w545, "Max Voltage"=w613, "error out 3"=w585, "f"=w591, "SampClk.Rate"=w602, "error in (no error)"=w601, "drive_amplitude"=w567, "task in"=w586, "drive_freq"=w528, "volt_div"=w568) -> ("task out 4"=w599:refnum<k21>, "Array"=→"Waveform Graph":dbl[][], "CC read error"=→"CC read error":errorcluster, "Refnum out"=w579:refnum<k21>, 21:"error out"=→"error out":errorcluster, "error out 4"=w598:errorcluster, "error out 2"=w578:errorcluster, "Pirani pressure (mbar)"=→"Pirani pressure (mbar)":string, "CC pressure (mbar)"=→"CC pressure (mbar)":string, "Temps (C):"=→"Temps (C):":dbl[], 27:"error out"=→"Pirani read error":errorcluster)  [unwired: 5 in]
            n114 = call <vilib>:"DAQmx Stop Task.vi"("task/channels in"=w599, "error in"=w598) -> ("task out"=w605:refnum<k21>, "error out"=w604:errorcluster)  [unwired: 12 in]
            n115 = call <vilib>:"DAQmx Stop Task.vi"("task/channels in"=w579, "error in"=w578) -> ("task out"=w582:refnum<k21>, "error out"=w581:errorcluster)  [unwired: 12 in]
            n116 = call <vilib>:"DAQmx Wait Until Done.vi"("task/channels in"=w549, "timeout (sec)"=10.0, "error in"=w548) -> ("task out"=w554:refnum<k21>, "error out"=w550:errorcluster)  [unwired: 11 in]
            n117 = call <vilib>:"DAQmx Clear Task.vi"("task in"=w605, "error in"=w604) -> ("error out"=w606:errorcluster)  [unwired: 13 in]
            n118 = call <vilib>:"DAQmx Clear Task.vi"("task in"=w582, "error in"=w581) -> ("error out"=w583:errorcluster)  [unwired: 13 in]
            n119 = call <vilib>:"DAQmx Stop Task.vi"("task/channels in"=w554, "error in"=w550) -> ("task out"=w555:refnum<k21>, "error out"=w551:errorcluster)  [unwired: 12 in]
            n120 = call <vilib>:"DAQmx Clear Task.vi"("task in"=w555, "error in"=w551) -> ("error out"=w553:errorcluster)  [unwired: 13 in]
            n121 = call <vilib>:"Simple Error Handler.vi"("type of dialog (OK msg:1)"=w603, "error in (no error)"=w606) -> ()  [unwired: 3 in, 5 out]
            n122 = call <vilib>:"Simple Error Handler.vi"("type of dialog (OK msg:1)"=w580, "error in (no error)"=w583) -> ()  [unwired: 3 in, 5 out]
            n123 = call <vilib>:"Simple Error Handler.vi"("type of dialog (OK msg:1)"=w552, "error in (no error)"=w553) -> ()  [unwired: 3 in, 5 out]
            n124 = call "Time Delay"("Delay Time (s)"="Delay time between files(s)") -> ()  [unwired: 10 in, 1 out]
          }
        }
      }
    }
  }
  n125 = case shown="True" "Use interferometer" {
    frame False {
    }
    frame True {
      w788 = FALSE ("Move")
      w794 = 0
      n126 = Bundle(FALSE, 0, "") -> (w800:errorcluster)  [unwired: 1 in]
      n127 = call <userlib>:"port init.vi"("SerialPort (1)"="Controller Serial Port") -> ("Visa Handle"=w796:refnum<visa-resource-name>)  [unwired: 3 in, 1 out]
      n128 = local write "Manual Move"(w788) -> ()
      n129 = call "enter / leave remote mode.vi"("error in"=w800, "enter / disable remote mode (True)"=TRUE, "VISA handle in"=w796) -> ("error out"=w797:errorcluster, "VISA handle out"=w798:refnum<visa-resource-name>, "TimeoutFlag"=w799:bool)  [unwired: 6 in]
      n130 = local write "Auto Move"(w788) -> ()
      n131 = local write "Timeout"(w799) -> ()
      n132 = call <vilib>:"Initialize.vi"("Serial Port"="Arduino Serial Port", "Error In"="Error In") -> ("Error Out"=w808:errorcluster, "Device Name"=→"Device Name":string, "LINX Ref"=w809:T5)  [unwired: 7 in]
      n133 = local write "Stop Button"(FALSE ("Stop Button")) -> ()
      n134 = while {
        tunnel: w798 -> [w841]
        shift-right: [w840] -> _
        shift-left: w794 -> [w842]
        shift-right: [w833] -> w791
        shift-left: w797 -> [w834]
        tunnel: [w836] -> w792
        tunnel: [w837] -> w790
        shift-right: [w839] -> _
        shift-left: w794 -> [w838]
        tunnel: [w835] -> w789
        tunnel: "Jog during auto" -> [w829]
        stop <- w830 stop-if-true
        n135 = case shown="False" w829 {
          tunnel: w842 -> [w851 w946]
          tunnel: w841 -> [w853 w944]
          tunnel: [w850 w942] -> w840
          tunnel: [w851 w934] -> w839
          tunnel: w838 -> [w850 w933]
          tunnel: [w852 w925] -> w837
          tunnel: [2 ("Axis out") w924] -> w836
          tunnel: [w849 w918] -> w835
          tunnel: w834 -> [w858 w916]
          tunnel: [w857 w909] -> w833
          tunnel: [w845 w909] -> w831
          tunnel: "Auto Move" -> [w844 w908]
          tunnel: "Auto Motion Direction" -> [w843 w907]
          tunnel: "Move Period (ms)" -> [w846 _]
          frame True {
            n136 = Select(t=1 ("Jog mode"), s=w843, f=-1 ("Jog mode")) -> (s? t:f=w854:i32)
            n137 = case shown="True" w844 {
              tunnel: w858 -> [w859 w874]
              tunnel: [w859 w873] -> w857
              tunnel: w854 -> [_ w872]
              tunnel: w853 -> [w861 w871]
              tunnel: [w861 w870] -> w852
              tunnel: [w860 w865] -> w849
              tunnel: u32 1 ("Axis in") -> [w860 w869]
              tunnel: w846 -> [_ w868]
              tunnel: [w859 w864] -> w845
              tunnel: w844 -> [_ w863]
              tunnel: w843 -> [_ w862]
              frame False {
              }
              frame True {
                n138 = flat-sequence {
                  tunnel: w874 -> [w887]
                  tunnel: w872 -> [w885]
                  tunnel: w871 -> [w884]
                  tunnel: [w886] -> w878
                  tunnel: [w883] -> w877
                  tunnel: w869 -> [w882]
                  tunnel: [w881] -> w866
                  tunnel: w863 -> [w880]
                  tunnel: w862 -> [w879]
                  tunnel: w878 -> [w891]
                  tunnel: w877 -> [w890]
                  tunnel: [w891] -> w876
                  tunnel: [w890] -> w875
                  tunnel: w868 -> [w889]
                  tunnel: [w888] -> w867
                  tunnel: w866 -> [w888]
                  tunnel: [w902] -> w870
                  tunnel: [w900] -> w873
                  tunnel: w876 -> [w905]
                  tunnel: w875 -> [w906]
                  tunnel: w867 -> [w904]
                  tunnel: [w901] -> w865
                  tunnel: [w900] -> w864
                  frame #0 {
                    n139 = local write "Motion Direction Indicator"(w879) -> ()
                    n140 = local write "Move Indicator"(w880) -> ()
                    n141 = call <userlib>:"Move jog.vi"("error in"=w887, "Jog mode"=w885, "Axis in"=w882, "VISA Handle in"=w884) -> ("error out"=w886:errorcluster, "Axis out"=w881:i32, "VISA Handle out"=w883:refnum<visa-resource-name>)  [unwired: 2 in, 1 out]
                  }
                  frame #1 {
                    n142 = while {
                      tunnel: w889 -> [w898]
                      stop <- w894 stop-if-true
                      n143 = local read "Stop Button"() -> (w897:bool)
                      n144 = local read "Auto Move"() -> (w893:bool)
                      n145 = local read "Stop Movement"() -> (w895:bool)
                      n146 = Not(x=w893) -> (.not. x?=w892:bool)
                      n147 = Or(x=w892, y=w897) -> (x .or. y?=w896:bool)
                      n148 = Or(x=w896, y=w895) -> (x .or. y?=w894:bool)
                      n149 = Wait Until Next ms Multiple(millisecond multiple=w898) -> ()  [unwired: 1 out]
                    }
                  }
                  frame #2 {
                    n150 = local write "Move Indicator"(FALSE ("Move Indicator")) -> ()
                    n151 = call <userlib>:"Move jog.vi"("error in"=w905, "Jog mode"=0, "Axis in"=w904, "VISA Handle in"=w906) -> ("error out"=w900:errorcluster, "Axis out"=w901:i32, "VISA Handle out"=w902:refnum<visa-resource-name>)  [unwired: 2 in, 1 out]
                  }
                }
              }
            }
          }
          frame False {
            n152 = Not Equal?(x="Positive Move Steps", y=w946) -> (x != y?=w947:bool)
            n153 = Not Equal?(x="Negative Move Steps", y=w933) -> (x != y?=w930:bool)
            n154 = case shown="True" w908 {
              selector: w908 -> [_ w951]
              tunnel: ["Motion Direction" w950] -> w936
              tunnel: ["Manual Move" w951] -> w915
              tunnel: w907 -> [_ w950]
              frame False {
              }
              frame True {
              }
            }
            "Move Indicator" <- w915
            "Motion Direction Indicator" <- w936
            n155 = Or(x=w947, y=w930) -> (x .or. y?=w931:bool)
            n156 = case shown="True" w931 {
              tunnel: w916 -> [w1036 w1050]
              tunnel: w944 -> [w1035 w1048]
              tunnel: 1 ("Axis in") -> [w1033 w1041]
              tunnel: "Positive Move Steps" -> [_ w1042]
              tunnel: [w1037 w1042] -> w943
              tunnel: w946 -> [w1037 _]
              tunnel: [w1036 w1046] -> w940
              tunnel: [w1035 w1045] -> w941
              tunnel: "Negative Move Steps" -> [_ w1039]
              tunnel: [w1034 w1039] -> w935
              tunnel: w933 -> [w1034 _]
              tunnel: [w1033 w1038] -> w929
              frame False {
              }
              frame True {
                n157 = call <userlib>:"set positive step size.vi"("error in"=w1050, "Step size (positive direction)"=w1042, "Axis in"=w1041, "VISA Handle in"=w1048) -> ("error out"=w1047:errorcluster, "Axis out"=w1043:i32, "VISA Handle out"=w1044:refnum<visa-resource-name>, "TimeoutFlag"=w1049:bool)  [unwired: 2 in]
                n158 = local write "Timeout"(w1049) -> ()
                n159 = call <userlib>:"set negative step size.vi"("error in"=w1047, "Step size (negative direction)"=w1039, "Axis in"=w1043, "VISA Handle in"=w1044) -> ("error out"=w1046:errorcluster, "Axis out"=w1038:i32, "VISA Handle out"=w1045:refnum<visa-resource-name>, "TimeoutFlag"=w1040:bool)  [unwired: 2 in]
                n160 = local write "Timeout"(w1040) -> ()
              }
            }
            n161 = Select(t=1 ("Number of steps"), s=w936, f=-1) -> (s? t:f=w937:i32)
            n162 = Compound Arithmetic op=AND("Move Slide  2", invert "Move Slide Back 3") -> (w910:bool)
            n163 = Compound Arithmetic op=AND("Move Slide Back 3", invert "Move Slide  2") -> (w911:bool)
            n164 = case shown="False" w915 {
              tunnel: w943 -> [w992 w1028]
              tunnel: [w992 w1028] -> w942
              tunnel: w941 -> [w988 w1029]
              tunnel: [w987 w1030] -> w926
              tunnel: w940 -> [w989 w1032]
              tunnel: [w986 w1031] -> w927
              tunnel: w937 -> [_ w1027]
              tunnel: w935 -> [w991 w1026]
              tunnel: [w991 w1026] -> w934
              tunnel: [w990 w1024] -> w924
              tunnel: w929 -> [w990 w1023]
              tunnel: "Slide Jog Speed 2" -> [w984 _]
              tunnel: w911 -> [w983 _]
              tunnel: w910 -> [w982 _]
              frame False {
                n165 = case shown="False" w982 {
                  tunnel: w989 -> [w998 w1022]
                  tunnel: [w997 w1021] -> w986
                  tunnel: w988 -> [w996 w1020]
                  tunnel: [w995 w1019] -> w987
                  tunnel: w984 -> [w1000 w1018]
                  tunnel: w983 -> [w999 _]
                  tunnel: [w993 w1017] -> _
                  tunnel: u32 1 ("Axis in") -> [w994 w1016]
                  frame False {
                    n166 = case shown="True" w999 {
                      tunnel: w1000 -> [_ w1015]
                      tunnel: w998 -> [w1001 w1013]
                      tunnel: [w1002 w1012] -> w997
                      tunnel: w996 -> [w1004 w1011]
                      tunnel: [w1003 w1010] -> w995
                      tunnel: w994 -> [w1007 w1009]
                      tunnel: [w1005 w1008] -> w993
                      frame False {
                        n167 = call <userlib>:"Move jog.vi"("error in"=w1001, "Jog mode"=0, "Axis in"=w1007, "VISA Handle in"=w1004) -> ("error out"=w1002:errorcluster, "Axis out"=w1005:i32, "VISA Handle out"=w1003:refnum<visa-resource-name>)  [unwired: 2 in, 1 out]
                      }
                      frame True {
                        n168 = Negate(x=w1015) -> (-x=w1014:i32)
                        n169 = call <userlib>:"Move jog.vi"("error in"=w1013, "Jog mode"=w1014, "Axis in"=w1009, "VISA Handle in"=w1011) -> ("error out"=w1012:errorcluster, "Axis out"=w1008:i32, "VISA Handle out"=w1010:refnum<visa-resource-name>)  [unwired: 2 in, 1 out]
                      }
                    }
                  }
                  frame True {
                    n170 = call <userlib>:"Move jog.vi"("error in"=w1022, "Jog mode"=w1018, "Axis in"=w1016, "VISA Handle in"=w1020) -> ("error out"=w1021:errorcluster, "Axis out"=w1017:i32, "VISA Handle out"=w1019:refnum<visa-resource-name>)  [unwired: 2 in, 1 out]
                  }
                }
              }
              frame True {
                n171 = call <userlib>:"move relative.vi"("error in"=w1032, "Number of steps"=w1027, "Axis in"=w1023, "VISA Handle in"=w1029) -> ("error out"=w1031:errorcluster, "Axis out"=w1024:i32, "VISA Handle out"=w1030:refnum<visa-resource-name>, "TimeoutFlag"=w1025:bool)  [unwired: 2 in]
                n172 = local write "Timeout"(w1025) -> ()
              }
            }
            n173 = Compound Arithmetic op=AND("Move Slide", invert "Move Slide Back") -> (w922:bool)
            n174 = Compound Arithmetic op=AND("Move Slide Back", invert "Move Slide") -> (w920:bool)
            n175 = case shown="False" w922 {
              tunnel: w927 -> [w957 w981]
              tunnel: [w956 w980] -> w909
              tunnel: w926 -> [w955 w979]
              tunnel: [w954 w978] -> w925
              tunnel: "Slide Jog Speed" -> [w959 w977]
              tunnel: w920 -> [w958 _]
              tunnel: [w952 w976] -> w918
              tunnel: u32 2 ("Axis in") -> [w953 w975]
              frame False {
                n176 = case shown="False" w958 {
                  tunnel: w959 -> [_ w974]
                  tunnel: w957 -> [w960 w972]
                  tunnel: [w961 w971] -> w956
                  tunnel: w955 -> [w963 w970]
                  tunnel: [w962 w969] -> w954
                  tunnel: w953 -> [w966 w968]
                  tunnel: [w964 w967] -> w952
                  frame False {
                    n177 = call <userlib>:"Move jog.vi"("error in"=w960, "Jog mode"=0, "Axis in"=w966, "VISA Handle in"=w963) -> ("error out"=w961:errorcluster, "Axis out"=w964:i32, "VISA Handle out"=w962:refnum<visa-resource-name>)  [unwired: 2 in, 1 out]
                  }
                  frame True {
                    n178 = Negate(x=w974) -> (-x=w973:i32)
                    n179 = call <userlib>:"Move jog.vi"("error in"=w972, "Jog mode"=w973, "Axis in"=w968, "VISA Handle in"=w970) -> ("error out"=w971:errorcluster, "Axis out"=w967:i32, "VISA Handle out"=w969:refnum<visa-resource-name>)  [unwired: 2 in, 1 out]
                  }
                }
              }
              frame True {
                n180 = call <userlib>:"Move jog.vi"("error in"=w981, "Jog mode"=w977, "Axis in"=w975, "VISA Handle in"=w979) -> ("error out"=w980:errorcluster, "Axis out"=w976:i32, "VISA Handle out"=w978:refnum<visa-resource-name>)  [unwired: 2 in, 1 out]
              }
            }
          }
        }
        n181 = Wait Until Next ms Multiple(millisecond multiple="Move Period (ms)") -> ()  [unwired: 1 out]
        n182 = Or(x="Stop Button", y=w831) -> (x .or. y?=w830:bool)
      }
      n183 = while {
        tunnel: w809 -> [w1089]
        tunnel: [w1088] -> w785
        tunnel: [w1054] -> w786
        tunnel: w808 -> [w1087]
        shift-right: [w1068] -> _
        shift-left: 0.0 ("Displacement") -> [w1060]
        shift-right: [w1069] -> _
        shift-left: _ -> [w1070]
        shift-right: [w1064] -> _
        shift-left: _ -> [w1062]
        stop <- w1056 stop-if-true
        w1083 = 200.0 ("sampling freq: fs")
        n184 = local read "Motion Direction Indicator"() -> (w1061:bool)
        n185 = call-poly <vilib>:"Analog Read.vi"("Error In"=w1087, "Analog Channel"="Analog Channel", "LINX Resource"=w1089) -> ("Error Out"=w1054:errorcluster, "AI Value"=w1076:dbl, "LINX Resource"=w1088:T5)  [unwired: 5 in, 1 out]
        "Raw Signal" <- w1076
        n186 = local read "Move Indicator"() -> (w1071:bool)
        n187 = Select(t=0.0, s="Zero", f=w1060) -> (s? t:f=w1059:dbl)
        n188 = call <vilib>:"Butterworth Filter PtByPt.vi"("initialize"="initialize", "order"="order", "filter type"="filter type", "low cutoff freq: fl"="low cutoff freq: fl", "high cutoff freq: fh"="high cutoff freq: fh", "sampling freq: fs"=w1083, "x"=w1076) -> ("Filtered x"=w1066:dbl)  [unwired: 2 in, 1 out]
        "Filtered Signal" <- w1066
        n189 = Exclusive Or(1:w1061, 2:w1062) -> (0:w1063:bool)
        n190 = Not(x=w1071) -> (.not. x?=w1072:bool)
        n191 = local read "Stop Button"() -> (w1055:bool)
        n192 = Or(x=w1072, y=w1063) -> (x .or. y?=w1051:bool)
        "Reset Fringe Counter" <- w1051
        n193 = call "Measure Fringe Displacement Simple.vi"("Photodiode Output"=w1066, "Fringe Counter Settings"="Fringe Counter Settings", "Reset"=w1051) -> ("Displacement"=w1069:dbl, "Input Signals"=→"Input Signals" →"Main Sig":dbl[][], "Stepped Signal"=→"Stepped Signal":dbl, "Output Signal"=→"Fringe Counter Output Signal":dbl[])  [unwired: 8 in, 1 out]
        "Relative Displacement" <- w1069
        n194 = case shown="True" w1071 {
          tunnel: w1059 -> [w1091 w1099]
          tunnel: [w1091 w1100] -> w1068
          tunnel: w1070 -> [_ w1095]
          tunnel: w1069 -> [_ w1097]
          tunnel: w1061 -> [w1090 w1096]
          tunnel: [w1090 w1096] -> w1064
          tunnel: w1051 -> [_ w1093]
          frame False {
          }
          frame True {
            n195 = Select(t=0.0, s=w1093, f=w1095) -> (s? t:f=w1094:dbl)
            n196 = Subtract(x=w1097, y=w1094) -> (x-y=w1098:dbl)
            n197 = case shown="False" w1096 {
              tunnel: [w1103 w1106] -> w1100
              tunnel: w1099 -> [w1101 w1105]
              tunnel: w1098 -> [w1102 w1104]
              frame False {
                n198 = Subtract(x=w1101, y=w1102) -> (x-y=w1103:dbl)
              }
              frame True {
                n199 = Add(x=w1105, y=w1104) -> (x+y=w1106:dbl)
              }
            }
          }
        }
        n200 = Or(x=w1054, y=w1055) -> (x .or. y?=w1056:bool)
        n201 = Reciprocal(x=w1083) -> (1/x=w1081:dbl)
        n202 = Multiply(x=1000.0 ("y"), y=w1081) -> (x*y=w1080:dbl)
        n203 = To Unsigned Long Integer(number=w1080) -> (unsigned 32bit integer=w1079:u32)
        n204 = Multiply(x=1000000.0, y=w1068) -> (x*y=→"Displacement" →"Total Displacement" →"Main Output":dbl)
        n205 = Wait Until Next ms Multiple(millisecond multiple=w1079) -> ()  [unwired: 1 out]
      }
      n206 = flat-sequence {
        tunnel: w792 -> [w818]
        tunnel: w791 -> [w817]
        tunnel: w790 -> [w816]
        tunnel: w789 -> [w813]
        tunnel: w786 -> [w811]
        tunnel: w785 -> [w810]
        frame #0 {
          n207 = call <userlib>:"stop motion.vi"("error in"=w817, "Axis in"=w818, "VISA Handle in"=w816) -> ("error out"=w815:errorcluster, "VISA Handle out"=w814:refnum<visa-resource-name>)  [unwired: 3 in, 2 out]
          n208 = call <userlib>:"Close.vi"("Error In"=w811, "LINX Resource"=w810) -> ("Error Out"=w812:errorcluster)  [unwired: 8 in, 1 out]
          n209 = call <vilib>:"Simple Error Handler.vi"("error in (no error)"=w812) -> ()  [unwired: 4 in, 5 out]
          n210 = call <userlib>:"stop motion.vi"("error in"=w815, "Axis in"=w813, "VISA Handle in"=w814) -> ("error out"=w825:errorcluster, "VISA Handle out"=w819:refnum<visa-resource-name>, "TimeoutFlag"=w822:bool)  [unwired: 3 in, 1 out]
          n211 = local write "Timeout"(w822) -> ()
          n212 = call "enter / leave remote mode.vi"("error in"=w825, "enter / disable remote mode (True)"=FALSE, "VISA handle in"=w819) -> ("error out"=w821:errorcluster, "VISA handle out"=w820:refnum<visa-resource-name>, "TimeoutFlag"=→"Timeout":bool)  [unwired: 6 in]
          n213 = call <userlib>:"close.vi"("VISA Handle in"=w820) -> ()  [unwired: 4 in, 1 out]
          n214 = call <vilib>:"General Error Handler.vi"("error in (no error)"=w821) -> ()  [unwired: 10 in, 5 out]
        }
        frame #1 {
          n215 = Stop() -> ()  [unwired: 1 in]
        }
      }
    }
  }
  n216 = case shown="True" w12 {
    tunnel: w16 -> [_ w1108]
    tunnel: w15 -> [_ w1107]
    frame False {
    }
    frame True {
      w1112 = 56 items=["No Error", "Argument Error", "Memory Full", "Out of Zone", "End of File", "File Already Open", "Generic File IO Error", "File Not Found", "File Permission Error", "Disk Full", "Duplicate Path", "Too Many Files Open", "Not Enabled", "Resource File Not Found", "Cannot Add Resource", "Resource Not Found", "Image Not Found", "Image Memory Error", "Pen Does Not Exist", "Config Bad Type", "Config Token Not Found", "Config Parse Error", "Config Memory Error", "Bad External Code Format", "Bad External Code Offset", "External Code Not Present", "Null Window", "Destroy Window Mixup", "Null Menu", "Print Aborted", "Bad Print Record", "Print Driver Error", "Windows Error During Print", "Memory Error During Print", "Print Dialog Error", "Generic Print Error", "Invalid Device Refnum", "Device Not Found", "Device Parameter Error", "Device Unit Error", "Can't Open Device", "Device Call Aborted", "Generic Error", "Cancelled By User", "Object ID Too Low", "Object ID Too High", "Object Not In Heap", "Unknown Heap", "Bad DefProc ID", "DefProc Not In Table", "Message Out Of Range", "Null Method", "Unknown Message", "Manager Call Not Supported", "Bad address", "Connection In progress", "Connection timed out", "Connection is already in progress", "Network attribute not supported", "Network error", "Address in use", "System out of memory", "Connection aborted", "Connection refused", "Connection is not connected", "Connection is already connected", "Connection closed", "Initialize error (interapplication manager)", "Bad occurrence", "Wait on unbound occurrence handler", "Occurrence queue overflow", "Bad path", "Semaphore not signaled", "Unrecognized type (interapplication manager)"] ("2nd Error to Convert")
      w1111 = 62 items=["No Error", "Argument Error", "Memory Full", "Out of Zone", "End of File", "File Already Open", "Generic File IO Error", "File Not Found", "File Permission Error", "Disk Full", "Duplicate Path", "Too Many Files Open", "Not Enabled", "Resource File Not Found", "Cannot Add Resource", "Resource Not Found", "Image Not Found", "Image Memory Error", "Pen Does Not Exist", "Config Bad Type", "Config Token Not Found", "Config Parse Error", "Config Memory Error", "Bad External Code Format", "Bad External Code Offset", "External Code Not Present", "Null Window", "Destroy Window Mixup", "Null Menu", "Print Aborted", "Bad Print Record", "Print Driver Error", "Windows Error During Print", "Memory Error During Print", "Print Dialog Error", "Generic Print Error", "Invalid Device Refnum", "Device Not Found", "Device Parameter Error", "Device Unit Error", "Can't Open Device", "Device Call Aborted", "Generic Error", "Cancelled By User", "Object ID Too Low", "Object ID Too High", "Object Not In Heap", "Unknown Heap", "Bad DefProc ID", "DefProc Not In Table", "Message Out Of Range", "Null Method", "Unknown Message", "Manager Call Not Supported", "Bad address", "Connection In progress", "Connection timed out", "Connection is already in progress", "Network attribute not supported", "Network error", "Address in use", "System out of memory", "Connection aborted", "Connection refused", "Connection is not connected", "Connection is already connected", "Connection closed", "Initialize error (interapplication manager)", "Bad occurrence", "Wait on unbound occurrence handler", "Occurrence queue overflow", "Bad path", "Semaphore not signaled", "Unrecognized type (interapplication manager)"] ("1st Error to Convert")
      n217 = TCP Close Connection(connection ID=w1107, error in (no error)=w1108) -> (error out=w1109:errorcluster)  [unwired: 1 in, 1 out]
      n218 = call <vilib>:"Error to Warning.vi"("1st Error to Convert"=w1111, "2nd Error to Convert"=w1112, "error in"=w1109) -> ("warning out"=w1110:errorcluster)  [unwired: 12 in]
      n219 = call <vilib>:"Simple Error Handler.vi"("error in (no error)"=w1110) -> ()  [unwired: 4 in, 5 out]
    }
  }
  n220 = case shown="True" w5 {
    tunnel: w7 -> [_ w1123]
    tunnel: w6 -> [_ w1122]
    frame False {
    }
    frame True {
      n221 = call <vilib>:"ag33xxx - Config Waveform.vi"("VISA session"=w1122, "Offset (0.00 V)"=0.0, "Frequency (1000 Hz)"=1000.0, "Amplitude (0.1 Vpp)"=1.0, "error in (no error)"=w1123) -> ("dup VISA session"=w1115:refnum<visa-resource-name>, "error out"=w1117:errorcluster)  [unwired: 9 in]
      n222 = call <vilib>:"ag33xxx - Error Query.vi"("error in (no error)"=w1117, "VISA session"=w1115) -> ("error out"=w1118:errorcluster, "dup VISA session"=w1119:refnum<visa-resource-name>)  [unwired: 6 in, 2 out]
      n223 = call <vilib>:"ag33xxx - Error Message.vi"("VISA session"=w1119, "error in (no error)"=w1118) -> ("dup VISA session"=w1114:refnum<visa-resource-name>, "error out"=w1116:errorcluster)  [unwired: 9 in, 3 out]
      n224 = call <vilib>:"ag33xxx - Close.vi"("error in (no error)"=w1116, "VISA session"=w1114) -> ()  [unwired: 9 in, 1 out]
    }
  }
